vi "UDPSingleReceiveBestPhil3.vi"(5 "expectedRepetitions":i32=10, 8 "error in (no error)":errorcluster, 9 "Boolean":bool, 10 "Timeout":i32=4000) -> (0 "error out":errorcluster, 1 "Data Received":string, 2 "# of Bytes Received":i32, 6 "packets read":i32=1024)   [LabVIEW 2014]
uses:
  GlobComm.vi
panel:
  out "String Length":u32
  out "voidcounter":dbl
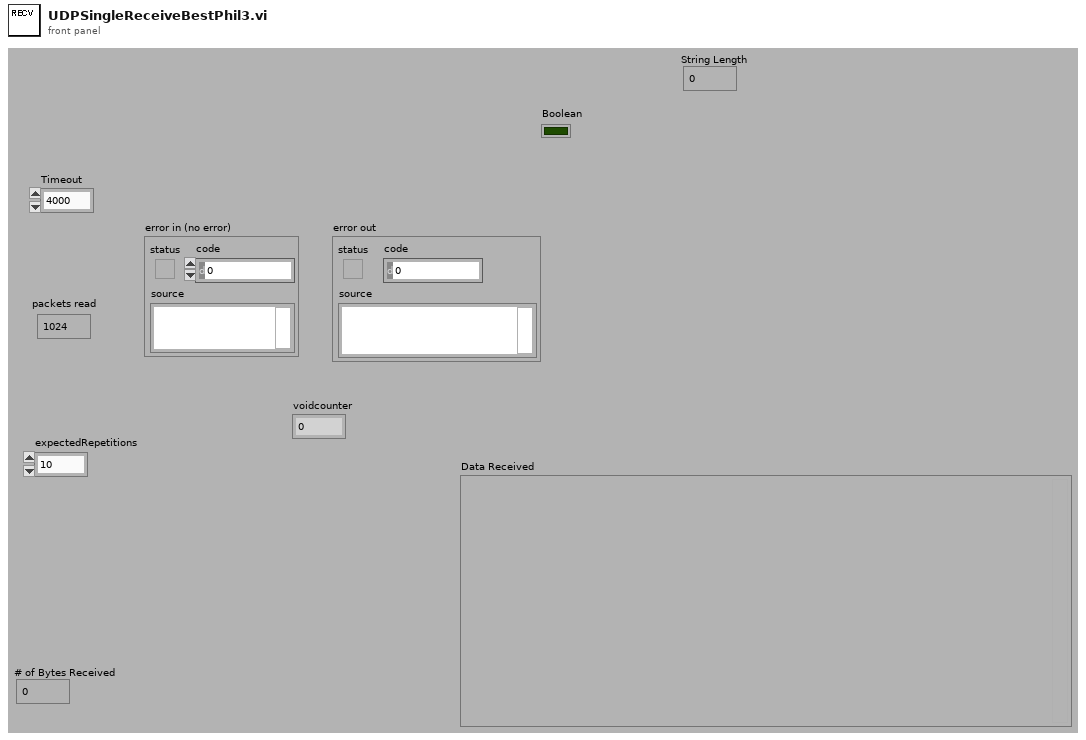
[diagram p1: front panel]
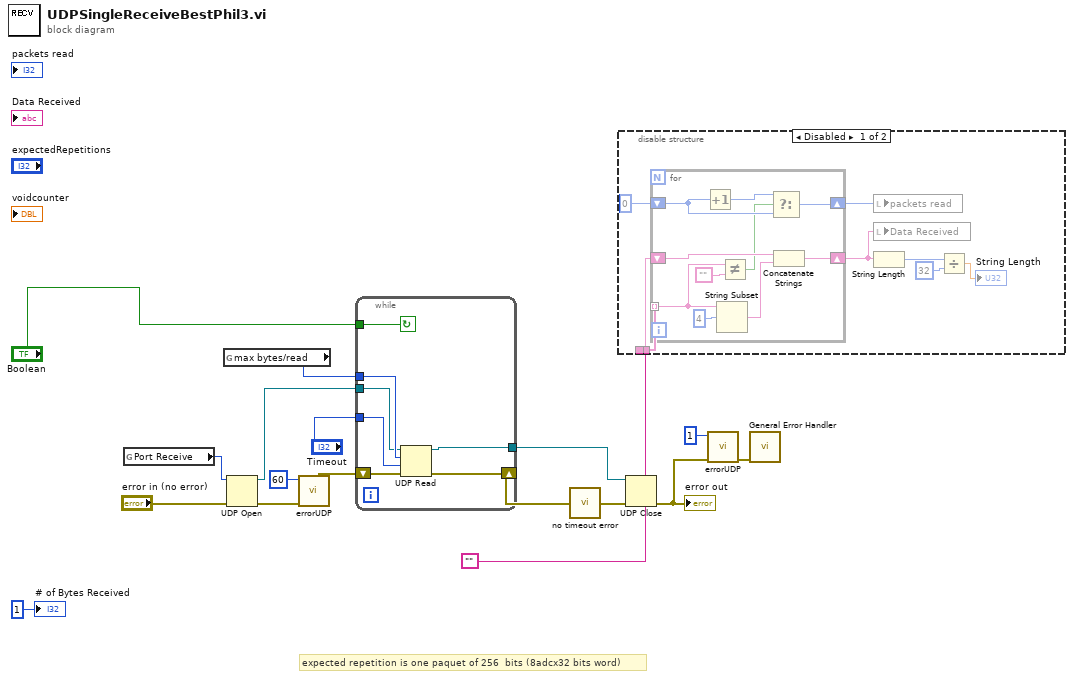
[diagram p0: block diagram]
diagram:
  # "expected repetition is one paquet of 256  bits (8adcx32 bits word)"
  n1 = global read "GlobComm.vi" "Port Receive"() -> (w5:u16)
  n2 = global read "GlobComm.vi" "max bytes/read"() -> (w4:i32)
  n3 = UDP Open(8:"error in (no error)", 11:w5) -> (port=w15:refnum<k16>, 0:w12:errorcluster)  [unwired: 4 out]
  n4 = call "errorUDP.vi"("error in (no error) 2"=w12, "errorcode"=60) -> ("error out 2"=w11:errorcluster)  [unwired: 9 out]
  n5 = while {
    tunnel: w4 -> [w24]
    tunnel: "Timeout" -> [w23]
    tunnel: w15 -> [w20]
    tunnel: [w22] -> w13
    shift-right: [w19] -> w16
    shift-left: w11 -> [w21]
    tunnel: "Boolean" -> [w18]
    stop <- w18 continue-if-true
    n6 = UDP Read(connection ID=w20, max size (548)=w24, timeout ms (25000)=w23, 8:w21) -> (error out=w19:errorcluster, 3:w22:refnum<k16>)  [unwired: 3 out]
  }
  n7 = call "no timeout error.vi"("error in (no error)"=w16) -> ("error out"=w14:errorcluster)
  n8 = disable-structure shown="Disabled" {
    disable-tunnel: "" -> [w32 _]
    disable-tunnel: _ -> [w31 _]
    frame Disabled {
      n9 = for {
        tunnel: w31 -> [w37] mode=indexing
        shift-right: [w42] -> w30
        shift-left: w32 -> [w41]
        shift-right: [w36] -> w25
        shift-left: 0 -> [w34]
        n10 = Increment(x=w34) -> (x+1=w35:i32)
        n11 = String Subset(string=w37, offset (0)=4) -> (substring=w39:string)  [unwired: 1 out]
        n12 = Not Equal?(x=w37, y="") -> (x != y?=w33:bool)
        n13 = Select(t=w35, s=w33, f=w34) -> (s? t:f=w36:i32)
        n14 = Concatenate Strings(w41, w39) -> (w42:string)
      }
      n15 = local write "packets read"(w25) -> ()
      n16 = local write "Data Received"(w30) -> ()
      n17 = String Length(string=w30) -> (length=w29:i32)
      n18 = Divide(x=w29, y=32) -> (x/y=→"String Length":dbl)
    }
    frame Enabled {
    }
  }
  n19 = UDP Close(connection ID=w13, 8:w14) -> (error out=w9:errorcluster)  [unwired: 1 out]
  "error out" <- w9
  n20 = call "errorUDP.vi"("error in (no error) 2"=w9, "errorcode"=1) -> ("error out 2"=w8:errorcluster)  [unwired: 9 out]
  n21 = call <vilib>:"General Error Handler.vi"("error in (no error)"=w8) -> ()  [unwired: 2 in, 13 out]
  "# of Bytes Received" <- 1
